vi "Y1.vi"(8 "error in (no error)":errorcluster, 11 "MagSpec_Bella in":refnum<class "MagSpec_Bella.lvclass">) -> (0 "error out":errorcluster, 3 "MagSpec_Bella out":refnum<class "MagSpec_Bella.lvclass">)   [LabVIEW 2013, in "MagSpec_Bella.lvclass"]
uses:
  MagSpec_Bella.lvclass
  MagSpec_Bella.lvclass/MagSpec_Bella.ctl
  <vilib>/gmath/NI_Gmath.lvlib
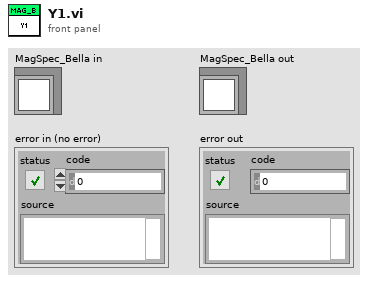
[diagram p1: front panel]
types:
  T1 = typedef "Calibration_Pixel_based.ctl" = cluster{"y1(pixel)":dbl[], "y2(pixel)":dbl[], "dp/B [MeV/C/B] (pixel)":dbl[], "energyDependence Input(pixel)":dbl[], "bending angle [deg](pixel)":dbl[], "total path(pixel)":dbl[], "pixel angle (y)(pixel)":dbl[], "energy dependence (pixel)":dbl[], "charge compensation (pixel)":dbl[], "Momentum [MeV/C](pixel)":dbl[], "angular compensation(pixel)":dbl[]}
  T2 = typedef "finalCalib--Cluster.ctl" = cluster{"X":dbl[][], "xi":dbl[][], "delta momentum":dbl, "Y":dbl[][], "yi":dbl[][], "angle (Y)":dbl[], "delta angle":dbl, "scale delta angle":dbl, "intraX":dbl, "intraY":dbl, "mask":dbl[][]}
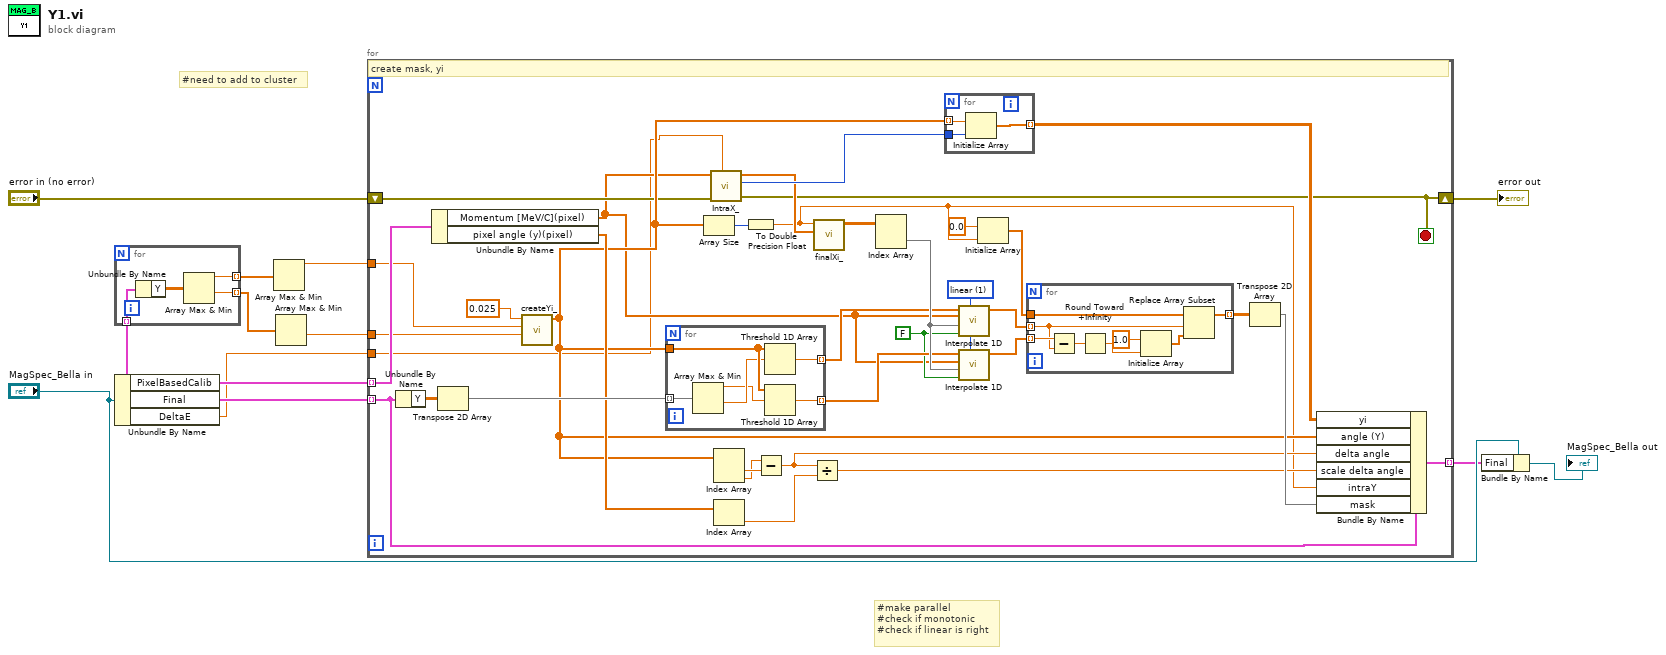
[diagram p0: block diagram]
diagram:
  # "#need to add to cluster"
  # "#make parallel\n#check if monotonic\n#check if linear is right"
  n1 = Unbundle By Name("MagSpec_Bella in") -> ("PixelBasedCalib"=w7:T1[], "Final"=w6:T2[], "DeltaE"=w1:dbl)
  n2 = for {
    tunnel: w6 -> [w16] mode=indexing
    tunnel: [w14] -> w5 mode=indexing
    tunnel: [w13] -> w4 mode=indexing
    n3 = Unbundle By Name(w16) -> ("Y"=w15:dbl[][])
    n4 = Array Max & Min(array=w15) -> (max value=w14:dbl, min value=w13:dbl)  [unwired: 2 out]
  }
  n5 = Array Max & Min(array=w5) -> (max value=w3:dbl)  [unwired: 3 out]
  n6 = Array Max & Min(array=w4) -> (min value=w2:dbl)  [unwired: 3 out]
  n7 = for {
    tunnel: w7 -> [w27] mode=indexing
    tunnel: w6 -> [w26] mode=indexing
    tunnel: [w25] -> w8 mode=indexing
    shift-right: [w23] -> w12
    shift-left: "error in (no error)" -> [w24]
    tunnel: w2 -> [w22]
    tunnel: w3 -> [w21]
    tunnel: w1 -> [w17]
    stop <- w23 stop-if-true
    w32 = FALSE ("X is monotonic")
    w33 = 1 items=["nearest", "linear", "spline", "cubic Hermite", "Lagrange"] ("method")
    # "create mask, yi"
    n8 = Unbundle By Name(w26) -> ("Y"=w28:dbl[][])
    n9 = Unbundle By Name(w27) -> ("Momentum [MeV/C](pixel)"=w20:dbl[], "pixel angle (y)(pixel)"=w36:dbl[])
    n10 = Transpose 2D Array(2D array=w28) -> (transposed array=w43:dbl[][])
    n11 = call "createYi_.vi"("Min"=w22, "Max"=w21, "delta"=0.025) -> ("Array"=w34:dbl[])  [unwired: 7 in, 1 out]
    n12 = for {
      tunnel: w43 -> [w66] mode=indexing
      tunnel: [w64] -> w44 mode=indexing
      tunnel: [w63] -> w45 mode=indexing
      tunnel: w34 -> [w65]
      n13 = Array Max & Min(array=w66) -> (max value=w61:dbl, min value=w62:dbl)  [unwired: 2 out]
      n14 = Threshold 1D Array(2:w62, 3:w65) -> (0:w63:dbl)  [unwired: 1 in]
      n15 = Threshold 1D Array(2:w61, 3:w65) -> (0:w64:dbl)  [unwired: 1 in]
    }
    n16 = Array Size(array=w34) -> (size(s)=w19:i32)
    n17 = call "IntraX_.vi"("DeltaE"=w17, "error in (no error)"=w24, "Momentum [MeV/C](pixel)"=w20) -> ("error out"=w23:errorcluster, "IntraX"=w31:i32, "Ramp Pattern"=w29:dbl[])  [unwired: 5 in, 1 out]
    n18 = Index Array(array=w34) -> (element #1=w40:dbl, element #2=w39:dbl)  [unwired: 2 in]
    n19 = Index Array(array=w36) -> (element=w41:dbl)  [unwired: 1 in]
    n20 = To Double Precision Float(number=w19) -> (double precision float=w18:dbl)
    n21 = Subtract(x=w39, y=w40) -> (x-y=w38:dbl)
    n22 = Divide(x=w38, y=w41) -> (x/y=w37:dbl)
    n23 = call "finalXi_.vi"("Ramp Pattern"=w29, "intraY"=w18) -> ("Array"=w30:dbl[][])  [unwired: 9 in]
    n24 = Index Array(array=w30) -> (element=w52:dbl[])  [unwired: 2 in]
    n25 = for {
      tunnel: w34 -> [w69] mode=indexing
      tunnel: w31 -> [w68]
      tunnel: [w67] -> w42 mode=indexing
      n26 = Initialize Array(w69, w68) -> (w67:dbl[])
    }
    n27 = call <vilib>:"Interpolate 1D.vi"("method"=w33, "X is monotonic"=w32, "xi"=w52, "X"=w20, "Y"=w45) -> ("yi"=w48:dbl[])  [unwired: 4 in, 2 out]
    n28 = call <vilib>:"Interpolate 1D.vi"("method"=w33, "X is monotonic"=w32, "xi"=w52, "X"=w20, "Y"=w44) -> ("yi"=w49:dbl[])  [unwired: 4 in, 2 out]
    n29 = Initialize Array(0.0 ("element"), w18) -> (w47:dbl[])
    n30 = for {
      tunnel: w48 -> [w57] mode=indexing
      tunnel: w47 -> [w58]
      tunnel: w49 -> [w60] mode=indexing
      tunnel: [w56] -> w50 mode=indexing
      n31 = Subtract(x=w60, y=w57) -> (x-y=w59:dbl)
      n32 = Round Toward +Infinity(x=w59) -> (ceil(x): smallest int >= x=w54:dbl)
      n33 = Initialize Array(1.0 ("element"), w54) -> (w53:dbl[])
      n34 = Replace Array Subset(array=w58, new element=w53, index=w57) -> (w56:dbl[])
    }
    n35 = Transpose 2D Array(2D array=w50) -> (transposed array=w51:dbl[][])
    n36 = Bundle By Name(cluster=w26, "yi"=w42, "angle (Y)"=w34, "delta angle"=w38, "scale delta angle"=w37, "intraY"=w18, "mask"=w51) -> (w25:T2)
  }
  "error out" <- w12
  n37 = Bundle By Name(cluster="MagSpec_Bella in", "Final"=w8) -> (→"MagSpec_Bella out":refnum<class "MagSpec_Bella.lvclass">)
